vi "Read Headers.vi"(6 "Starting Buffer (None)":string, 8 "error in (no error)":errorcluster, 9 "Stream in":refnum<k5>, 11 "Request in":refnum<class "Request.lvclass">) -> (0 "error out":errorcluster, 1 "Stream out":refnum<k5>, 3 "Request out":refnum<class "Request.lvclass">, 5 "Bytes":i32)   [LabVIEW 2020, in "HTTP Utils.lvlib" / "Request.lvclass"]
uses:
  Request.lvclass
  Request.lvclass/Request.ctl
  Cookie/Cookie.lvclass
  Cookie Map.ctl
  HTTP Utils.lvlib
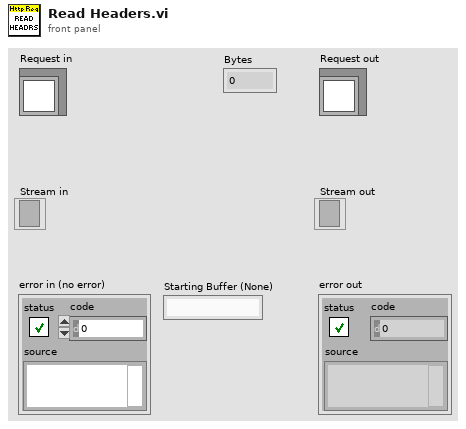
[diagram p1: front panel]
types:
  T1 = typedef "HTTP Utils.lvlib/Cookie Map.ctl" = map{string, refnum<class "Cookie.lvclass">}
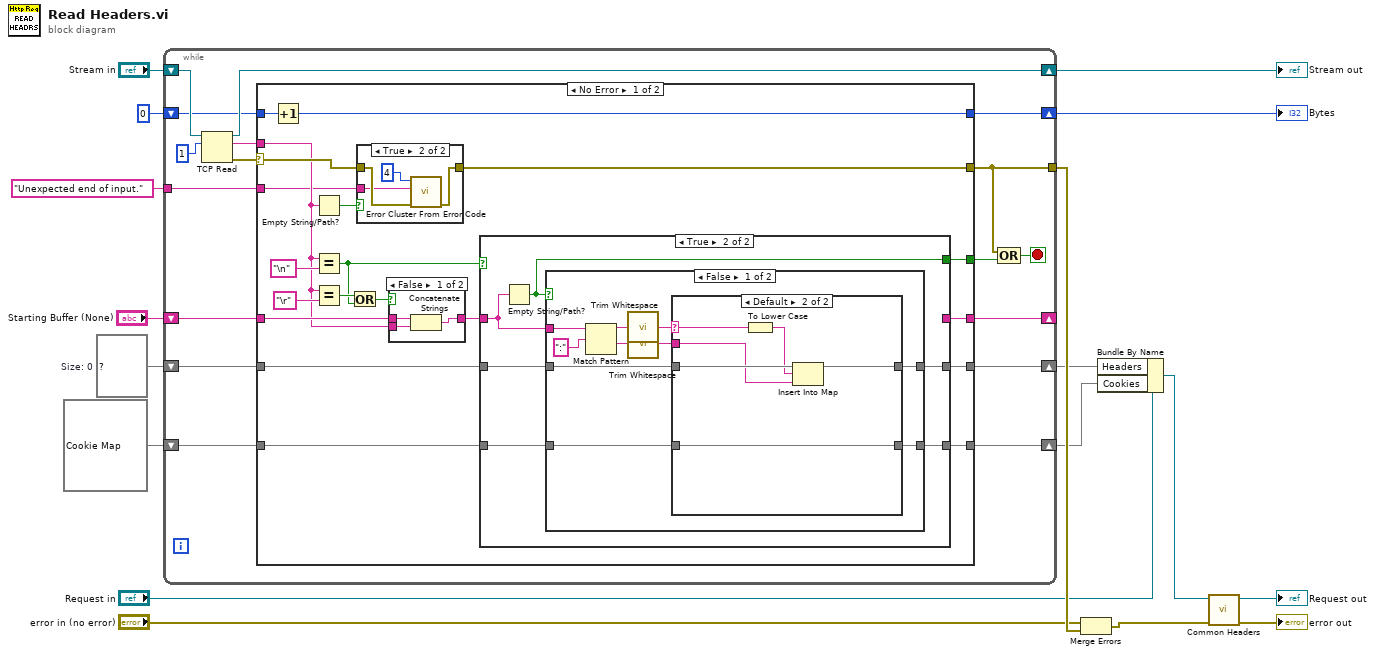
[diagram p0: block diagram]
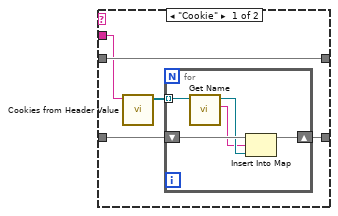
[diagram p4: hidden frame]
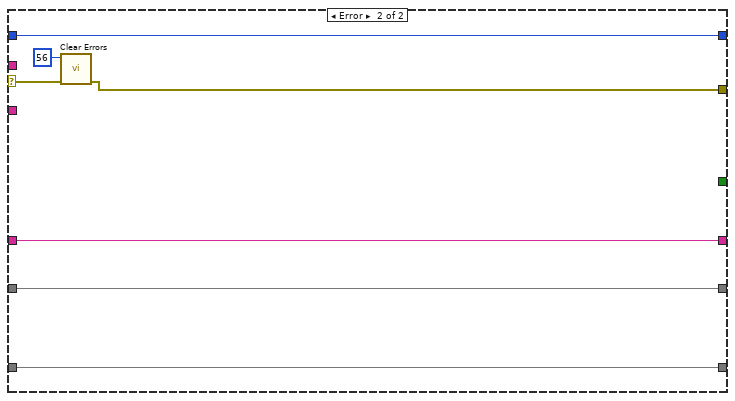
[diagram p7: hidden frame]
diagram:
  w12 = map{string, string} {}  # Size: 0
  n1 = while {
    shift-right: [w26] -> w10
    shift-left: "Stream in" -> [w33]
    shift-right: [w25] -> _
    shift-left: "Starting Buffer (None)" -> [w31]
    shift-right: [w29] -> w11
    shift-left: w12 -> [w30]
    tunnel: [w21] -> w17
    shift-right: [w24] -> w8
    shift-left: T1 {} ("Cookies") -> [w23]
    tunnel: "Unexpected end of input." -> [w20]
    shift-right: [w18] -> w1
    shift-left: 0 -> [w19]
    stop <- w27 stop-if-true
    n2 = TCP Read(connection ID=w33, bytes to read=1 ("Count")) -> (connection ID out=w26:refnum<k5>, data out=w22:string, error out=w34:errorcluster)  [unwired: 3 in]
    n3 = case shown="No Error" w34 {
      selector: w34 -> [w54 w104]
      tunnel: w31 -> [w49 w107]
      tunnel: w30 -> [w46 w106]
      tunnel: [w45 w106] -> w29
      tunnel: [w44 _] -> w28
      tunnel: [w43 w107] -> w25
      tunnel: [w42 w105] -> w24
      tunnel: w23 -> [w41 w105]
      tunnel: w22 -> [w40 _]
      tunnel: [w38 w102] -> w21
      tunnel: w20 -> [w37 _]
      tunnel: w19 -> [w36 w101]
      tunnel: [w35 w101] -> w18
      frame No Error {
        n4 = Increment(x=w36) -> (x+1=w35:i32)
        n5 = Empty String/Path?(string/path=w40) -> (empty?=w39:bool)
        n6 = Equal?(x=w40, y="\n") -> (x = y?=w47:bool)
        n7 = Equal?(x=w40, y="\r") -> (x = y?=w51:bool)
        n8 = Or(x=w51, y=w47) -> (x .or. y?=w50:bool)
        n9 = case shown="True" w39 {
          tunnel: w54 -> [w55 w57]
          tunnel: [w55 w59] -> w38
          tunnel: w37 -> [_ w56]
          frame False {
          }
          frame True {
            n10 = call <vilib>:"Error Cluster From Error Code.vi"("error in (no error)"=w57, "error message (\"\")"=w56, "error code (0)"=4) -> ("error out"=w59:errorcluster)  [unwired: 6 in]
          }
        }
        n11 = case shown="False" w50 {
          tunnel: w49 -> [w99 w100]
          tunnel: [w98 w100] -> w48
          tunnel: w40 -> [w97 _]
          frame False {
            n12 = Concatenate Strings(w99, w97) -> (w98:string)
          }
          frame True {
          }
        }
        n13 = case shown="True" w47 {
          tunnel: w48 -> [w61 w67]
          tunnel: w46 -> [w62 w66]
          tunnel: [w62 w65] -> w45
          tunnel: [_ w68] -> w44
          tunnel: [w61 _] -> w43
          tunnel: [w60 w64] -> w42
          tunnel: w41 -> [w60 w63]
          frame False {
          }
          frame True {
            n14 = Empty String/Path?(string/path=w67) -> (empty?=w68:bool)
            n15 = case shown="False" w68 {
              tunnel: w67 -> [w77 _]
              tunnel: w66 -> [w78 w96]
              tunnel: [w75 w96] -> w65
              tunnel: w63 -> [w70 w95]
              tunnel: [w69 w95] -> w64
              frame False {
                n16 = Match Pattern(string=w77, regular expression=":") -> (before substring=w74:string, after substring=w72:string)  [unwired: 1 in, 2 out]
                n17 = call <vilib>:"Trim Whitespace.vi"("string"=w74) -> ("trimmed string"=w73:string)  [unwired: 1 in]
                n18 = call <vilib>:"Trim Whitespace.vi"("string"=w72) -> ("trimmed string"=w71:string)  [unwired: 1 in]
                n19 = case shown="Default" w73 {
                  selector: w73 -> [_ w91]
                  tunnel: w78 -> [w83 w94]
                  tunnel: [w83 w92] -> w75
                  tunnel: w71 -> [w82 w90]
                  tunnel: w70 -> [w80 w89]
                  tunnel: [w79 w89] -> w69
                  frame "Cookie" {
                    n20 = call "Cookies from Header Value.vi"("Cookie Header Value"=w82) -> ("Cookies"=w81:refnum<class "Cookie.lvclass">[])  [unwired: 9 in, 1 out]
                    n21 = for {
                      tunnel: w81 -> [w88] mode=indexing
                      shift-right: [w84] -> w79
                      shift-left: w80 -> [w87]
                      n22 = call "Get Name.vi"("Cookie in"=w88) -> ("Name"=w85:string, "Cookie out"=w86:refnum<class "Cookie.lvclass">)  [unwired: 8 in, 1 out]
                      n23 = Insert Into Map(map in=w87, key=w85, value=w86) -> (map out=w84:T1)  [unwired: 2 out]
                    }
                  }
                  frame Default {
                    n24 = To Lower Case(string=w91) -> (all lower case string=w93:string)
                    n25 = Insert Into Map(map in=w94, key=w93, value=w90) -> (map out=w92:map{string, string})  [unwired: 2 out]
                  }
                }
              }
              frame True {
              }
            }
          }
        }
      }
      frame Error {
        n26 = call <vilib>:"Clear Errors.vi"("error in (no error)"=w104, "specific error code to clear (0: all)"=56) -> ("error out"=w102:errorcluster)  [unwired: 4 in, 1 out]
      }
    }
    n27 = Compound Arithmetic op=OR(w21, w28) -> (w27:bool)
  }
  "Stream out" <- w10
  "Bytes" <- w1
  n28 = Merge Errors("error in (no error)", w17) -> (w4:errorcluster)
  n29 = Bundle By Name(cluster="Request in", "Headers"=w11, "Cookies"=w8) -> (w6:refnum<class "Request.lvclass">)
  n30 = call "Common Headers.vi"("error in (no error)"=w4, "Request in"=w6) -> ("error out"=→"error out":errorcluster, "Request out"=→"Request out":refnum<class "Request.lvclass">)  [unwired: 8 in]
